vi "Set PDO transmit mapping.vi"(6 "PDO mapping":u32[](array[numeric]), 7 "timeout (1s)":dbl=1.0 min=0.0, 8 "error in (no error)":errorcluster, 9 "PDO channel":u8(ring) items=["PDO 1", "PDO 2", "PDO 3", "PDO 4"], 11 "SDO object in":refnum<k20>) -> (0 "error out":errorcluster, 1 "completion code":u32, 3 "SDO object out":refnum<k20>)   [LabVIEW 2016]
uses:
  <vilib>/CANopenLib/CANOPEN.llb/CANopen SDO Write [U32].vi
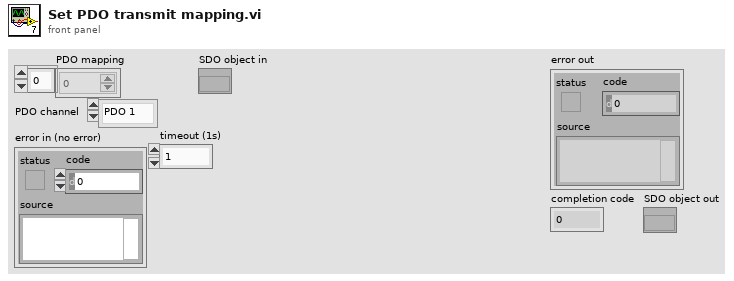
[diagram p1: front panel]
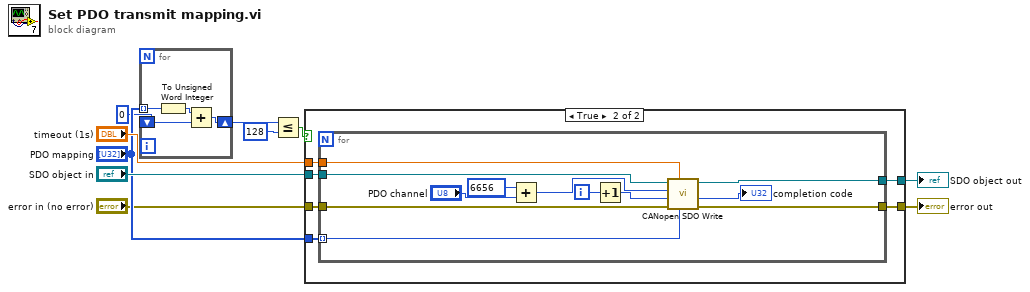
[diagram p0: block diagram]
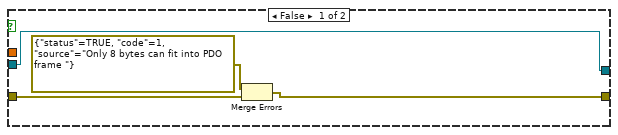
[diagram p2: hidden frame]
diagram:
  n1 = for {
    tunnel: "PDO mapping" -> [w13] mode=indexing
    shift-right: [w12] -> w5
    shift-left: u16 0 -> [w11]
    n2 = To Unsigned Word Integer(number=w13) -> (unsigned 16bit integer=w14:u16)
    n3 = Add(x=w14, y=w11) -> (x+y=w12:u16)
  }
  n4 = Less Or Equal?(x=w5, y=u16 128) -> (x <= y?=w3:bool)
  n5 = case shown="True" w3 {
    tunnel: "PDO mapping" -> [_ w24]
    tunnel: "timeout (1s)" -> [_ w23]
    tunnel: "SDO object in" -> [w16 w22]
    tunnel: [w16 w21] -> w8
    tunnel: [w17 w20] -> w7
    tunnel: "error in (no error)" -> [w15 w19]
    frame False {
      n6 = Merge Errors(errorcluster {"status"=TRUE, "code"=1, "source"="Only 8 bytes can fit into PDO frame "} ("error constant"), w15) -> (w17:errorcluster)
    }
    frame True {
      n7 = for {
        tunnel: w24 -> [w31] mode=indexing
        tunnel: w23 -> [w30]
        tunnel: w22 -> [w29]
        tunnel: [w28] -> w21
        tunnel: [w26] -> w20
        tunnel: w19 -> [w25]
        i -> [w33]
        n8 = Add(x=u16 6656, y="PDO channel") -> (x+y=w34:u16)
        n9 = Increment(x=w33) -> (x+1=w32:i32)
        n10 = call-poly <vilib>:"CANopen SDO Write.vi"("U32 data"=w31, "timeout (1s)"=w30, "error in (no error)"=w25, "object sub-index (0)"=w32, "object index"=w34, "SDO object in"=w29) -> ("error out"=w26:errorcluster, "completion code"=→"completion code":u32, "SDO object out"=w28:refnum<k20>)  [unwired: 3 in]
      }
    }
  }
  "error out" <- w7
  "SDO object out" <- w8
